vi "Sort file info metadata.vi"(0 "reference in":refnum<class "metadata.lvclass">, 5 "error in (no error)":errorcluster) -> (14 "reference out":refnum<class "metadata.lvclass">, 16 "file info":T1, 19 "error out":errorcluster)   [LabVIEW 2019, in "metadata.lvclass"]
uses:
  metadata.lvclass
  File info parameters.ctl
  Write time and date string --constant.ctl
  Read time and date string --constant.ctl
panel:
  out "Array":string[](array[string])
  out "Array 2":i32[](array[numeric])
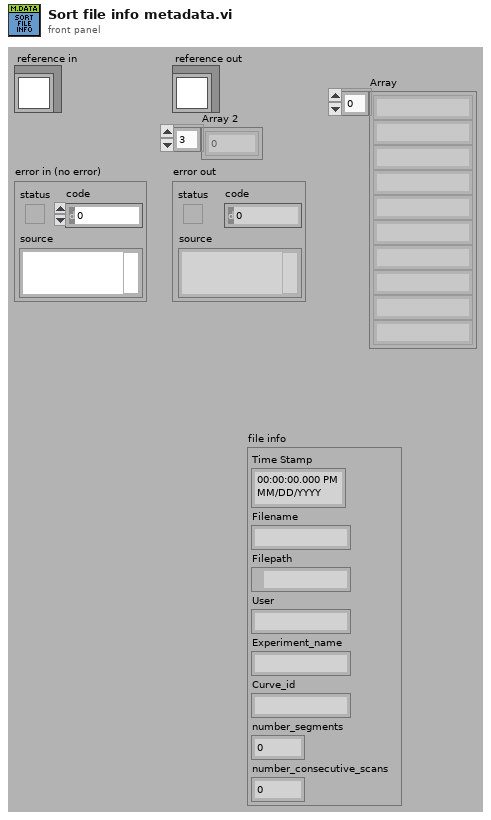
[diagram p1: front panel]
types:
  T1 = typedef "metadata.lvclass/File info parameters.ctl" = cluster{"Time Stamp":timestamp, "Filename":string, "Filepath":path, "User":string, "Experiment_name":string, "Curve_id":string, "number_segments":u8, "number_consecutive_scans":u32}
  T2 = typedef "metadata.lvclass/Read time and date string --constant.ctl" = string
  T3 = typedef "metadata.lvclass/Write time and date string --constant.ctl" = string
  T4 = typedef "metadata.lvclass/ObjectAttributesRef.ctl" = refnum<data-value>
  T5 = typedef "metadata.lvclass/ObjectAttributes.ctl" = cluster{"MyAttribute":dbl, "System Control":T6, "file info":T1, "Sample info":T7, "Cantilever info":T8, "XYZ piezos":T9, "Mapping":T10, "Fcurve segment":T11[], "Fast fpga segment":T13, "Chirp":T14, "precision (6)":i16, "width (-)":i16, "Metadata":T15, "config filepath":path, "Section names []":string[], "Property names []":string[], "nb elements":u16}
  T6 = typedef "metadata.lvclass/System control parameters.ctl" = cluster{"FPGA SW version":string, "TDMS file version":string, "Instrument":string, "Instrument model":string, "Instrument scanner":string, "Instrument clockrate (Mhz)":string, "Instrument tick time (us)":string}
  T7 = typedef "metadata.lvclass/Sample info parameters.ctl" = cluster{"Sample name":string, "Sample species":string}
  T8 = typedef "metadata.lvclass/Cantilever info parameters.ctl" = cluster{"spring constant calib method":string, "invOLS calib method":string, "thermal calib deflection channel":string, "model":string, "shape":string, "tip geometry":string, "Laser sum (V)":dbl, "Laser power (mA)":dbl, "invOLS_(nm/V)":dbl, "spring constant nominal (N/m)":dbl, "spring constant calib (N/m)":dbl, "resosnance frequency air calib (Hz)":dbl, "resosnance frequency calib (Hz)":dbl, "quality factor":dbl, "Acoefficident_GCI_(nN.s^1.3/m)":dbl, "half angle (deg)":dbl, "tip radius (m)":dbl, "tip height (m)":dbl, "system mount angle (deg)":dbl}
  T9 = typedef "metadata.lvclass/XYZ piezos parameters.ctl" = cluster{"X stage piezo sensitivity (nm/V)":dbl, "X stage piezo gain":dbl, "X velocity (V/tick)":dbl, "X closed loop":bool, "Y stage piezo sensitivity (nm/V)":dbl, "Y stage piezo gain":dbl, "Y velocity (V/tick)":dbl, "Y closed loop":bool, "Z stage piezo sensitivity (nm/V)":dbl, "Z stage piezo gain":dbl, "Z closed loop":bool, "X position (V)":dbl, "Y position (V)":dbl}
  T10 = typedef "metadata.lvclass/Mapping parameters.ctl" = cluster{"Mapping":bool, "index":u16, "position row":u16, "position column":u16, "next position row":i16, "next position column":i16, "X initial position (V)":dbl, "Y initial position (V)":dbl, "X step size (V)":dbl, "Y step size (V)":dbl}
  T11 = typedef "metadata.lvclass/Fcurve segment.ctl" = cluster{"type":T12, "fast_fpga_trigger":bool, "nb":u8, "duration (ticks)":i64, "nb points":i32, "sampling rate (S/s)":u32, "Zpiezo control out":string, "initial deflection (V)":dbl, "relative setpoint":bool, "setpoint on":bool, "setpoint (V)":dbl, "setpoint trigger channel":string, "velocity (V/tick)":dbl, "Z position setpoint trigger (V)":dbl, "Z retract length (V)":dbl, "dec factor":u32}
  T12 = typedef "metadata.lvclass/Segment type--combobox.ctl" = string
  T13 = typedef "metadata.lvclass/fast fpga segment parameters.ctl" = cluster{"Fast start time trigger":timestamp, "nb_points":u32, "sampling_rate_(S/s)":u32, "duration_(ticks)":u32}
  T14 = typedef "metadata.lvclass/Chirp added parameters.ctl" = cluster{"f start (Hz)":dbl, "f end (Hz)":dbl, "Sweep type":string}
  T15 = typedef "metadata.lvclass/Metadata output --cluster.ctl" = cluster{"Property Names":string[], "Property Values":variant[]}
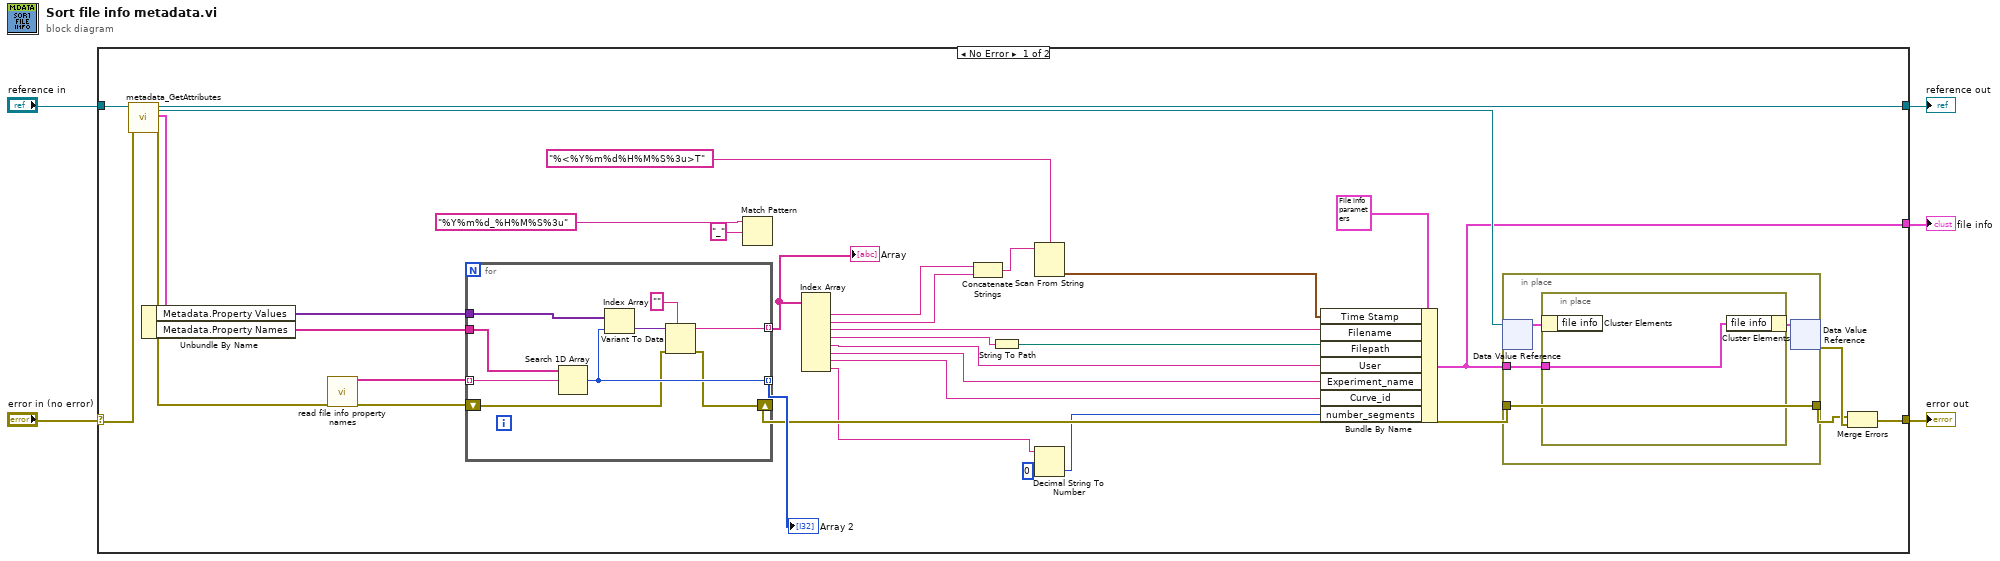
[diagram p0: block diagram]
diagram:
  n1 = case shown="No Error" "error in (no error)" {
    selector: "error in (no error)" -> [w35 w55]
    tunnel: [w39 w55] -> w4
    tunnel: [w34 w54] -> w2
    tunnel: "reference in" -> [w36 w54]
    tunnel: [w26 _] -> w1
    frame No Error {
      n2 = call "metadata_GetAttributes.vi"("reference in"=w36, "error in (no error)"=w35) -> ("reference out"=w34:refnum<class "metadata.lvclass">, "attributes ref"=w33:T4, "attributes"=w32:T5, "error out"=w24:errorcluster)  [unwired: 14 in]
      n3 = Unbundle By Name(w32) -> ("Metadata.Property Values"=w28:variant[], "Metadata.Property Names"=w31:string[])
      n4 = call "read file info property names.vi"("error in (no error)"=w24) -> ("Property names.File info"=w22:string[], "error out"=w23:errorcluster)  [unwired: 17 in]
      n5 = for {
        tunnel: w22 -> [w48] mode=indexing
        tunnel: [w45] -> w30 mode=indexing
        shift-right: [w41] -> w29
        shift-left: w23 -> [w42]
        tunnel: w31 -> [w47]
        tunnel: w28 -> [w46]
        tunnel: [w43] -> w27 mode=indexing
        n6 = Search 1D Array(1D array=w47, element=w48) -> (index of element=w45:i32)  [unwired: 1 in]
        n7 = Index Array(array=w46, index=w45) -> (element=w44:variant)
        n8 = Variant To Data(error in=w42, type="", Variant=w44) -> (data=w43:string, error out=w41:errorcluster)
      }
      "Array 2" <- w30
      "Array" <- w27
      n9 = Match Pattern(string=T3 "%Y%m%d_%H%M%S%3u" ("time format string (%c)"), regular expression="_") -> ()  [unwired: 1 in, 4 out]
      n10 = Index Array(array=w27) -> (element #1=w19:string, element #2=w18:string, element #3=w14:string, element #4=w13:string, element #5=w11:string, element #6=w10:string, element #7=w9:string, element #8=w7:string)  [unwired: 8 in]
      n11 = Concatenate Strings(w19, w18) -> (w17:string)
      n12 = String To Path(string=w13) -> (path=w12:path)
      n13 = Scan From String(format string=T2 "%<%Y%m%d%H%M%S%3u>T" ("time format string (%c)"), input string=w17) -> (output 1=w15:timestamp)  [unwired: 3 in, 3 out]
      n14 = Decimal String To Number(string=w7, default (0L)=u8 0 ("number_segments")) -> (number=w6:u8)  [unwired: 1 in, 1 out]
      n15 = Bundle By Name(cluster=T1 {"Time Stamp"=timestamp(0 s since 1904-01-01), "Filename"="", "Filepath"=path "", "User"="", "Experiment_name"="", "Curve_id"="", "number_segments"=0, "number_consecutive_scans"=0} ("file info"), "Time Stamp"=w15, "Filename"=w14, "Filepath"=w12, "User"=w11, "Experiment_name"=w10, "Curve_id"=w9, "number_segments"=w6) -> (w26:T1)
      n16 = in-place {
        in-place-border: w29 -> [w50]
        in-place-border: [w50] -> w37
        in-place-border: w26 -> [w49]
        n17 = in-place-dvr #1(w33) -> (w51:T5)  [unwired: 1 out]
        n18 = in-place {
          in-place-border: w49 -> [w53]
          n19 = in-place-cluster #2(w51) -> ()  [unwired: 1 out]
          n20 = in-place-cluster #2("file info"=w53) -> (w52:T5)
        }
        n21 = in-place-dvr #1(w52) -> (w38:errorcluster)  [unwired: 1 out]
      }
      n22 = Merge Errors(w37, w38) -> (w39:errorcluster)
    }
    frame Error {
    }
  }
  "error out" <- w4
  "reference out" <- w2
  "file info" <- w1
